vi "Get KeySight ENA Instrument Names.vi"(8 "error in (no error)":errorcluster, 11 "Semiconductor Module Context":T1) -> (0 "error out":errorcluster, 1 "Channel Lists":string[](array[string]), 2 "Instrument Names":string[](array[string]), 3 "Semiconductor Module Context Out":T1)   [LabVIEW 2013, in "ENA Custom Instrument.lvlib"]
uses:
  ENA Custom Instrument.lvlib
  <vilib>/NI_TestStand_SemiconductorModule/NI_TestStand_Semiconductor_Module.lvlibp/PinMap/General/SemiconductorModuleContext.ctl
  <vilib>/NI_TestStand_SemiconductorModule/NI_TestStand_Semiconductor_Module.lvlibp
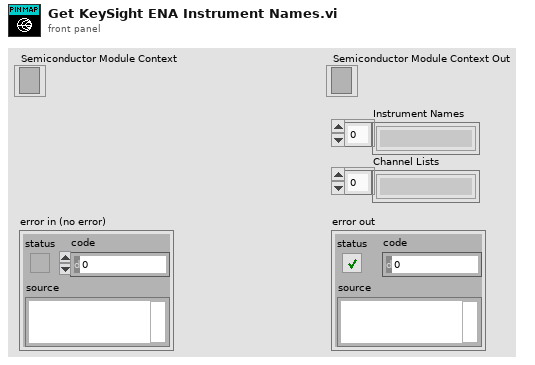
[diagram p1: front panel]
types:
  T1 = typedef "NI_TestStand_Semiconductor_Module.lvlibp/SemiconductorModuleContext.ctl" = refnum<k7>
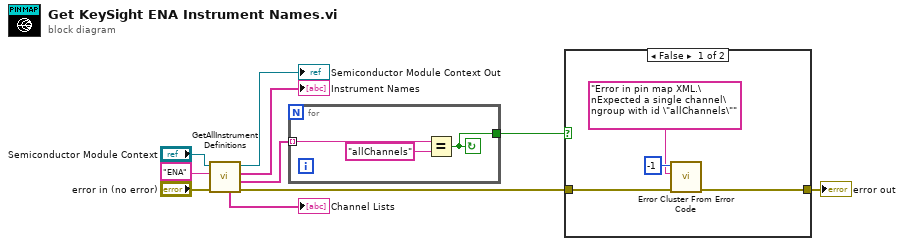
[diagram p0: block diagram]
diagram:
  n1 = call <vilib>:"GetAllInstrumentDefinitions.vi"("error in (no error)"="error in (no error)", "Instrument Type Id"="ENA", "Semiconductor Module Context"="Semiconductor Module Context") -> ("error out"=w2:errorcluster, "Channel Group Ids"=w6:string[], "Instrument Names"=→"Instrument Names":string[], "Semiconductor Module Context Out"=→"Semiconductor Module Context Out":T1, "Channel Lists"=→"Channel Lists":string[])  [unwired: 4 in]
  n2 = for {
    tunnel: w6 -> [w13] mode=indexing
    tunnel: [w11] -> w3
    stop <- w11 continue-if-true
    n3 = Equal?(x=w13, y="allChannels") -> (x = y?=w11:bool)
  }
  n4 = case shown="False" w3 {
    tunnel: w2 -> [w17 w18]
    tunnel: [w16 w18] -> w1
    frame False {
      n5 = call <vilib>:"Error Cluster From Error Code.vi"("error in (no error)"=w17, "error message (\"\")"="Error in pin map XML.\nExpected a single channel\ngroup with id \"allChannels\"" ("error message (\"\")"), "error code (0)"=-1) -> ("error out"=w16:errorcluster)  [unwired: 6 in]
    }
    frame True {
    }
  }
  "error out" <- w1
